vi "SVT UFF58 Write Record 6.vi"(0 "function refnum":refnum<k20>, 5 "DOF identification":T1={"function type"=enum."general or unknown", "function ID number"=0, "version number"=0, "load case ID number"=0, "response entity name"="NONE", "response node"=0, "response direction"=0, "reference entity name"="NONE", "reference node"=0, "reference direction"=0} {"reference direction" items=["-Z Rotation"=-6, "-Y Rotation"=-5, "-X Rotation"=-4, "-Z Translation"=-3, "-Y Translation"=-2, "-X Translation"=-1, "Scalar"=0, "+X Translation"=1, "+Y Translation"=2, "+Z Translation"=3, "+X Rotation"=4, "+Y Rotation"=5, "+Z Rotation"=6]; "response direction" items=["-Z Rotation"=-6, "-Y Rotation"=-5, "-X Rotation"=-4, "-Z Translation"=-3, "-Y Translation"=-2, "-X Translation"=-1, "Scalar"=0, "+X Translation"=1, "+Y Translation"=2, "+Z Translation"=3, "+X Rotation"=4, "+Y Rotation"=5, "+Z Rotation"=6]}, 11 "error in (no error)":errorcluster) -> (4 "dup function refnum":refnum<k20>, 15 "error out":errorcluster)   [LabVIEW 2017, in "SoundVib_UFF58.lvlib"]
doc: "Writes the values of the fields in record 6 of the UFF58 (universal file format) file. Record 6 contains the degree of freedom identification."
uses:
  <vilib>/addons/Sound and Vibration/svt_UFF58/SoundVib_UFF58.lvlib
  <vilib>/addons/Sound and Vibration/svt_UFF58/subVIs/sv_UFF58 DOF.ctl
  <vilib>/addons/Sound and Vibration/svt_UFF58/subVIs/sv_FunctionType.ctl
  <vilib>/addons/Sound and Vibration/svt_UFF58/subVIs/sv_UFF58 Response Direction.ctl
  <vilib>/Platform/storage/Storage.llb/Set Property (String).vi
  <vilib>/Platform/storage/Storage.llb/Set Property (I32).vi
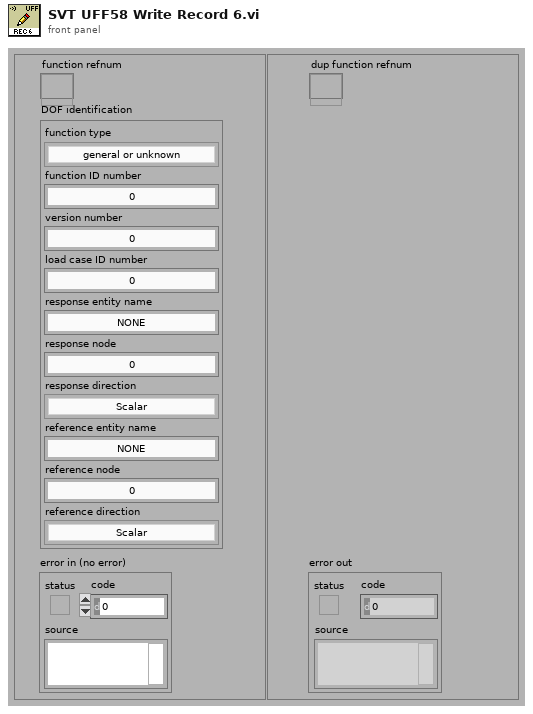
[diagram p1: front panel]
types:
  T1 = typedef "SoundVib_UFF58.lvlib/sv_UFF58 DOF.ctl" = cluster{"function type":T2, "function ID number":i32, "version number":i32, "load case ID number":i32, "response entity name":string, "response node":i32, "response direction":T3, "reference entity name":string, "reference node":i32, "reference direction":T3}
  T2 = typedef "SoundVib_UFF58.lvlib/sv_FunctionType.ctl" = enum16{"general or unknown", "time response", "auto spectrum", "cross spectrum", "frequency response function", "transmissibility", "coherence", "auto correlation", "cross correlation", "power spectral density (PSD)", "energy spectral density (ESD)", "probability density function", "spectrum", "cumulative frequency distribution", "peaks valley", "stress/cycles", "strain/cycles", "orbit", "mode indicator function", "force pattern", "partial power", "partial coherence", "eigenvalue", "eigenvector", "shock response spectrum", "finite impulse response filter", "multiple coherence", "order function", "phase compensation"}
  T3 = typedef "SoundVib_UFF58.lvlib/sv_UFF58 Response Direction.ctl" = i32
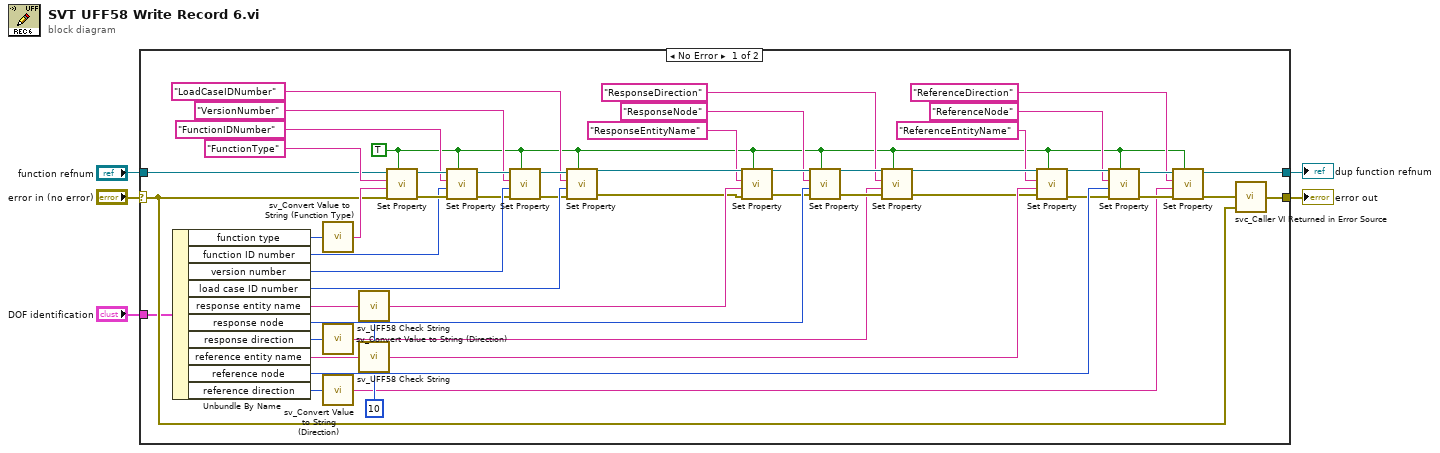
[diagram p0: block diagram]
diagram:
  n1 = case shown="No Error" "error in (no error)" {
    selector: "error in (no error)" -> [w12 w57]
    tunnel: "DOF identification" -> [w11 _]
    tunnel: [w13 w57] -> w4
    tunnel: [w49 w58] -> w1
    tunnel: "function refnum" -> [w48 w58]
    frame No Error {
      w10 = TRUE ("Create if not found (no:F)")
      w15 = 10 ("length (rest)")
      n2 = Unbundle By Name(w11) -> ("function type"=w45:T2, "function ID number"=w47:i32, "version number"=w46:i32, "load case ID number"=w43:i32, "response entity name"=w56:string, "response node"=w42:i32, "response direction"=w9:T3, "reference entity name"=w55:string, "reference node"=w41:i32, "reference direction"=w7:T3)
      n3 = call <vilib>:"sv_Convert Value to String (Function Type).vi"("function type"=w45) -> ("String"=w44:string)  [unwired: 14 in]
      n4 = call <vilib>:"sv_Convert Value to String (Direction).vi"("direction value"=w9) -> ("direction string"=w8:string)  [unwired: 14 in]
      n5 = call <vilib>:"sv_Convert Value to String (Direction).vi"("direction value"=w7) -> ("direction string"=w6:string)  [unwired: 14 in]
      n6 = call <vilib>:"sv_UFF58 Check String.vi"("field value"=w56, "field length"=w15) -> ("output string"=w51:string)  [unwired: 12 in, 1 out]
      n7 = call <vilib>:"sv_UFF58 Check String.vi"("field value"=w55, "field length"=w15) -> ("output string"=w50:string)  [unwired: 12 in, 1 out]
      n8 = call-poly <vilib>:"Set Property.vi"("Create if not found (no:F)"=w10, "error in (no error)"=w12, "Value"=w44, "Property name"="FunctionType", "storage refnum"=w48) -> ("error out"=w52:errorcluster, "storage refnum out"=w53:refnum<k20>)  [unwired: 5 in]
      n9 = call-poly <vilib>:"Set Property.vi"("Create if not found (no:F)"=w10, "error in (no error)"=w52, "Value"=w47, "Property name"="FunctionIDNumber", "storage refnum"=w53) -> ("error out"=w38:errorcluster, "storage refnum out"=w39:refnum<k20>)  [unwired: 5 in]
      n10 = call-poly <vilib>:"Set Property.vi"("Create if not found (no:F)"=w10, "error in (no error)"=w38, "Value"=w46, "Property name"="VersionNumber", "storage refnum"=w39) -> ("error out"=w35:errorcluster, "storage refnum out"=w36:refnum<k20>)  [unwired: 5 in]
      n11 = call-poly <vilib>:"Set Property.vi"("Create if not found (no:F)"=w10, "error in (no error)"=w35, "Value"=w43, "Property name"="LoadCaseIDNumber", "storage refnum"=w36) -> ("error out"=w31:errorcluster, "storage refnum out"=w33:refnum<k20>)  [unwired: 5 in]
      n12 = call-poly <vilib>:"Set Property.vi"("Create if not found (no:F)"=w10, "error in (no error)"=w31, "Value"=w51, "Property name"="ResponseEntityName", "storage refnum"=w33) -> ("error out"=w30:errorcluster, "storage refnum out"=w29:refnum<k20>)  [unwired: 5 in]
      n13 = call-poly <vilib>:"Set Property.vi"("Create if not found (no:F)"=w10, "error in (no error)"=w30, "Value"=w42, "Property name"="ResponseNode", "storage refnum"=w29) -> ("error out"=w26:errorcluster, "storage refnum out"=w27:refnum<k20>)  [unwired: 5 in]
      n14 = call-poly <vilib>:"Set Property.vi"("Create if not found (no:F)"=w10, "error in (no error)"=w26, "Value"=w8, "Property name"="ResponseDirection", "storage refnum"=w27) -> ("error out"=w24:errorcluster, "storage refnum out"=w23:refnum<k20>)  [unwired: 5 in]
      n15 = call-poly <vilib>:"Set Property.vi"("Create if not found (no:F)"=w10, "error in (no error)"=w24, "Value"=w50, "Property name"="ReferenceEntityName", "storage refnum"=w23) -> ("error out"=w21:errorcluster, "storage refnum out"=w22:refnum<k20>)  [unwired: 5 in]
      n16 = call-poly <vilib>:"Set Property.vi"("Create if not found (no:F)"=w10, "error in (no error)"=w21, "Value"=w41, "Property name"="ReferenceNode", "storage refnum"=w22) -> ("error out"=w17:errorcluster, "storage refnum out"=w19:refnum<k20>)  [unwired: 5 in]
      n17 = call-poly <vilib>:"Set Property.vi"("Create if not found (no:F)"=w10, "error in (no error)"=w17, "Value"=w6, "Property name"="ReferenceDirection", "storage refnum"=w19) -> ("error out"=w14:errorcluster, "storage refnum out"=w49:refnum<k20>)  [unwired: 5 in]
      n18 = call <vilib>:"svc_Caller VI Returned in Error Source.vi"("warning input to caller"=w12, "error in (no error)"=w14) -> ("error out"=w13:errorcluster)  [unwired: 3 in]
    }
    frame Error {
    }
  }
  "error out" <- w4
  "dup function refnum" <- w1
